vi "仪器参数设置.vi"(11 "仪器参数设置":T2 {"单位" items=["ug/L", "mg/L"]}) -> (3 "仪器参数设置输出":T1 {"单位" items=["ug/L", "mg/L"]})   [LabVIEW 2016, in "斯坦道CODMn.lvlib"]
uses:
  <vilib>/Utility/miscctls.llb/LVPointTypeDef.ctl
panel:
  in  "单位":enum16{"ug/L", "mg/L"}(ring)
  in  "标样校准时间":timestamp
  in  "二次多项式系数":dbl
  in  "线性相关系数":dbl
  in  "测量信号值":dbl
  in  "测量检出限":dbl
  in  "曲线斜率":dbl
  in  "曲线截距":dbl
  in  "空白校准时间":timestamp
  in  "消解时长":dbl
  in  "消解温度":dbl
  in  "测量间隔":dbl
  in  "测量精度":dbl
  in  "测量量程":dbl
  in  "取消":bool
  in  "确定":bool
  # "仪器参数设置"
  # "CODMn"
  # "监测参数"
  # "黑色框参数需要手动输入\n灰色框参数自动读取不需要手动输入"
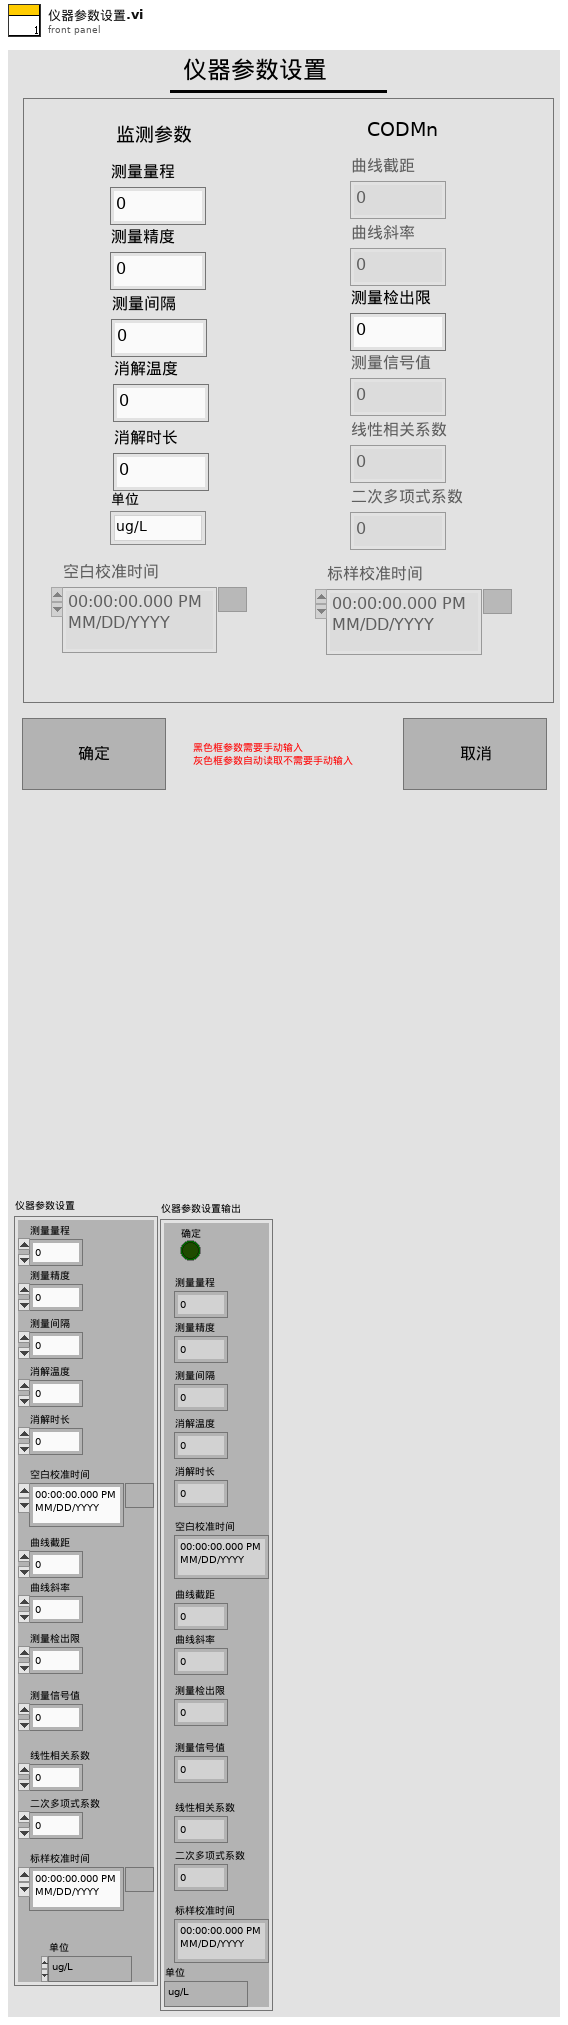
[diagram p1: front panel]
types:
  T1 = cluster{"确定":bool, "测量量程":dbl, "测量精度":dbl, "测量间隔":dbl, "消解温度":dbl, "消解时长":dbl, "空白校准时间":timestamp, "曲线截距":dbl, "曲线斜率":dbl, "测量检出限":dbl, "测量信号值":dbl, "线性相关系数":dbl, "二次多项式系数":dbl, "标样校准时间":timestamp, "单位":u16}
  T2 = cluster{"测量量程":dbl, "测量精度":dbl, "测量间隔":dbl, "消解温度":dbl, "消解时长":dbl, "空白校准时间":timestamp, "曲线截距":dbl, "曲线斜率":dbl, "测量检出限":dbl, "测量信号值":dbl, "线性相关系数":dbl, "二次多项式系数":dbl, "标样校准时间":timestamp, "单位":u16}
  T3 = typedef "LVPointTypeDef.ctl" = cluster{"Horizontal":i16, "Vertical":i16}
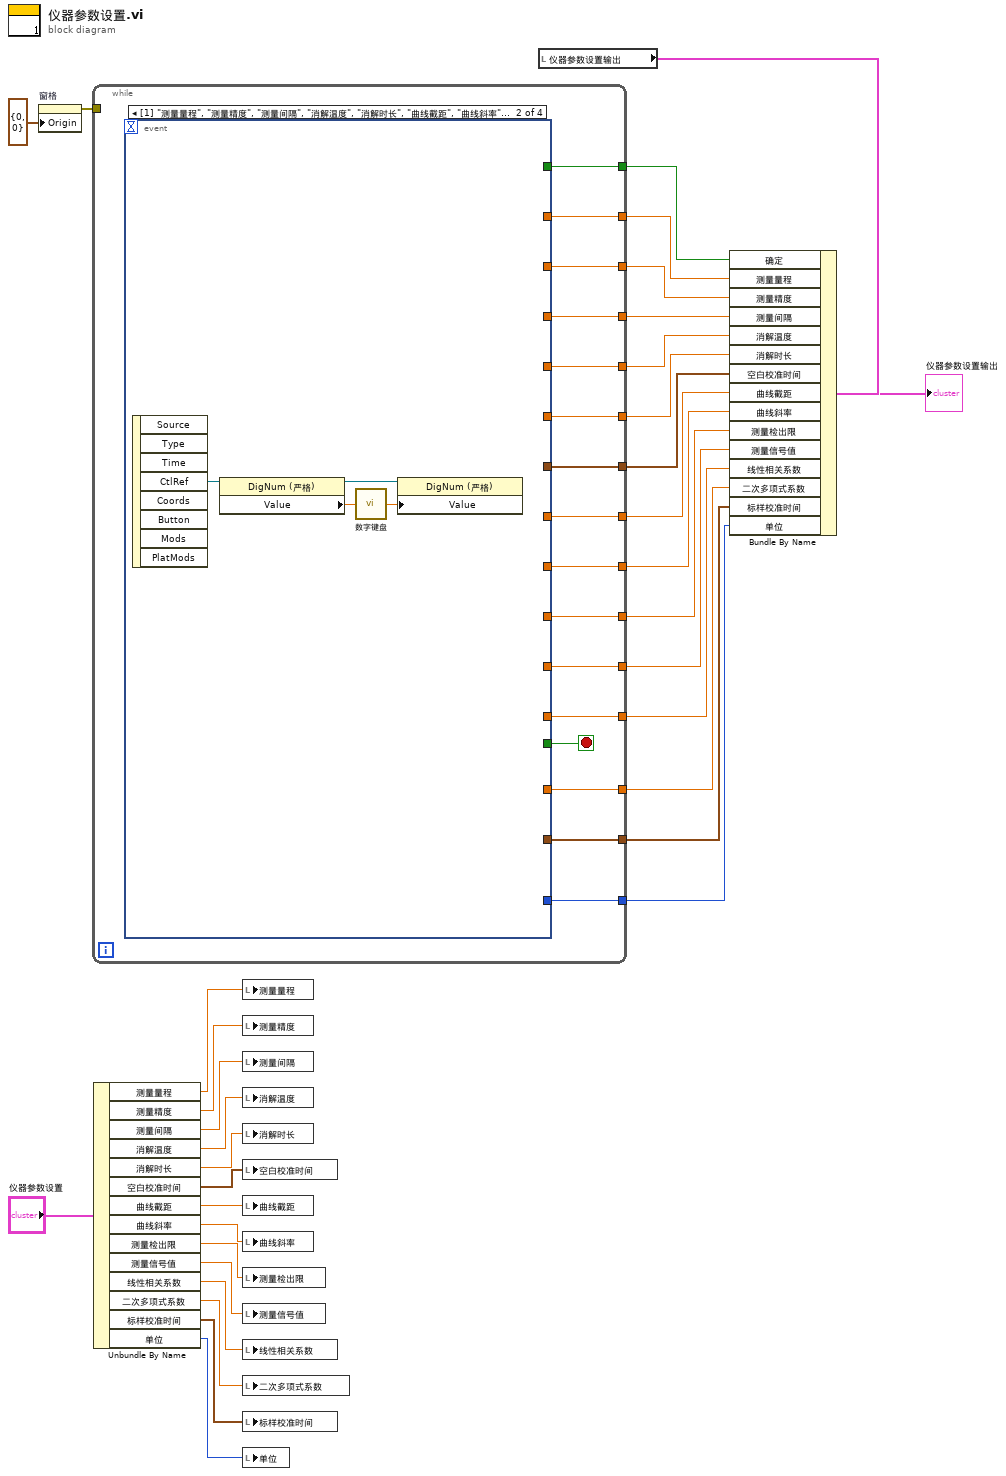
[diagram p0: block diagram]
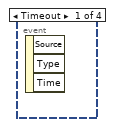
[diagram p2: hidden frame]
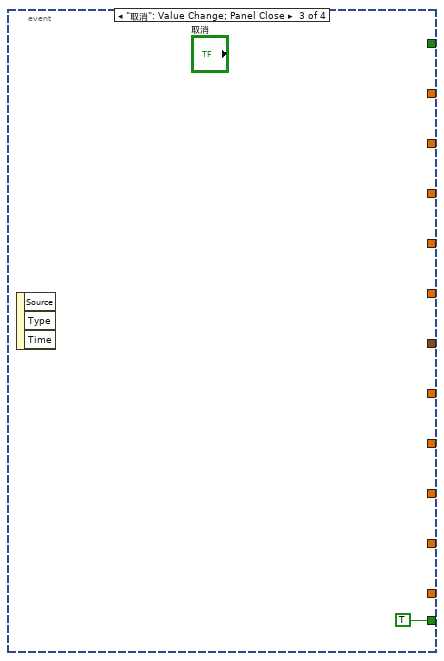
[diagram p3: hidden frame]
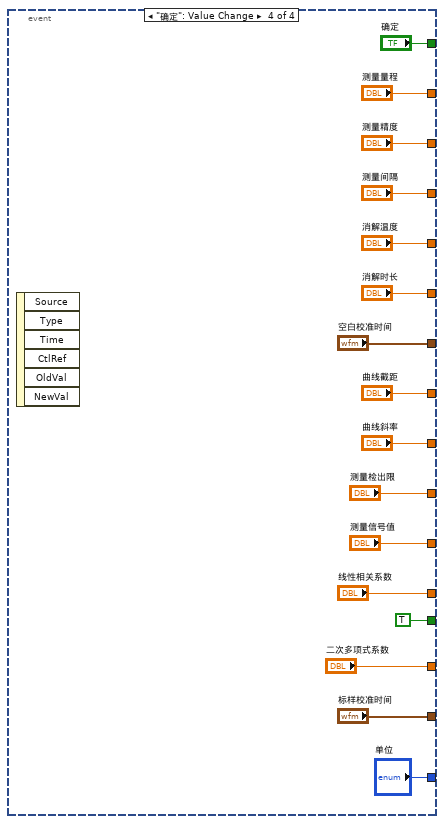
[diagram p4: hidden frame]
diagram:
  n1 = property on="窗格" class="Pane"("Origin"=T3 {"Horizontal"=0, "Vertical"=0} ("原点")) -> (error out=w33:errorcluster)  [unwired: 2 in, 1 out]
  n2 = while {
    tunnel: w33 -> [_]
    tunnel: [w49] -> w32
    tunnel: [w48] -> w28
    tunnel: [w47] -> w27
    tunnel: [w46] -> w26
    tunnel: [w45] -> w25
    tunnel: [w44] -> w24
    tunnel: [w43] -> w23
    tunnel: [w42] -> w22
    tunnel: [w41] -> w21
    tunnel: [w40] -> w20
    tunnel: [w39] -> w19
    tunnel: [w38] -> w18
    tunnel: [w37] -> w17
    tunnel: [w36] -> w16
    tunnel: [w35] -> w1
    stop <- w50 stop-if-true
    n3 = event shown="[1] \"测量量程\", \"测量精度\", \"测量间隔\", \"消解温度\", \"消解时长\", \"曲线截距\", \"曲线斜率\", \"测量检出限\", \"测量信号值\", \"线性相关系数\", \"二次多项式系数\": 鼠标按下" {
      selector: _ -> [_ _ _ _]
      dyn-events: _ -> [_ _ _ _]
      timeout: _ -> [_ _ _ _]
      tunnel: [_ _ TRUE TRUE] -> w50
      tunnel: [_ _ _ "确定"] -> w49
      tunnel: [_ _ _ "标样校准时间"] -> w48
      tunnel: [_ _ _ "二次多项式系数"] -> w47
      tunnel: [_ _ _ "线性相关系数"] -> w46
      tunnel: [_ _ _ "测量信号值"] -> w45
      tunnel: [_ _ _ "测量检出限"] -> w44
      tunnel: [_ _ _ "曲线斜率"] -> w43
      tunnel: [_ _ _ "曲线截距"] -> w42
      tunnel: [_ _ _ "空白校准时间"] -> w41
      tunnel: [_ _ _ "消解时长"] -> w40
      tunnel: [_ _ _ "消解温度"] -> w39
      tunnel: [_ _ _ "测量间隔"] -> w38
      tunnel: [_ _ _ "测量精度"] -> w37
      tunnel: [_ _ _ "测量量程"] -> w36
      tunnel: [_ _ _ "单位"] -> w35
      event Timeout {
        n4 = event-data() -> ()  [unwired: 1 in, 3 out]
      }
      event "测量量程", "测量精度", "测量间隔", "消解温度", "消解时长", "曲线截距", "曲线斜率", "测量检出限", "测量信号值", "线性相关系数", "二次多项式系数": Mouse Down {
        n5 = event-data() -> ("CtlRef"=w51:refnum<vi>)  [unwired: 1 in, 7 out]
        n6 = property class="DigNum (严格)"(reference=w51) -> (reference out=w53:refnum<vi>, "Value"=w54:dbl)  [unwired: 1 in, 1 out]
        n7 = call "数字键盘.vi"("OldNumber"=w54) -> ("NewNumber"=w52:sgl)
        n8 = property class="DigNum (严格)"(reference=w53, "Value"=w52) -> ()  [unwired: 1 in, 2 out]
      }
      event "取消": Value Change; Panel Close {
        n9 = event-data() -> ()  [unwired: 1 in, 3 out]
      }
      event "确定": Value Change {
        n10 = event-data() -> ()  [unwired: 1 in, 6 out]
      }
    }
  }
  n11 = Unbundle By Name("仪器参数设置") -> ("测量量程"=w15:dbl, "测量精度"=w14:dbl, "测量间隔"=w13:dbl, "消解温度"=w12:dbl, "消解时长"=w11:dbl, "空白校准时间"=w10:timestamp, "曲线截距"=w9:dbl, "曲线斜率"=w8:dbl, "测量检出限"=w7:dbl, "测量信号值"=w6:dbl, "线性相关系数"=w5:dbl, "二次多项式系数"=w4:dbl, "标样校准时间"=w3:timestamp, "单位"=w2:u16)
  n12 = local write "测量量程"(w15) -> ()
  n13 = local write "测量精度"(w14) -> ()
  n14 = local write "测量间隔"(w13) -> ()
  n15 = local write "消解温度"(w12) -> ()
  n16 = local write "消解时长"(w11) -> ()
  n17 = local write "空白校准时间"(w10) -> ()
  n18 = local write "曲线截距"(w9) -> ()
  n19 = local write "曲线斜率"(w8) -> ()
  n20 = local write "测量检出限"(w7) -> ()
  n21 = local write "测量信号值"(w6) -> ()
  n22 = local write "线性相关系数"(w5) -> ()
  n23 = local write "二次多项式系数"(w4) -> ()
  n24 = local write "标样校准时间"(w3) -> ()
  n25 = local write "单位"(w2) -> ()
  n26 = local read "仪器参数设置输出"() -> (w30:T1)
  n27 = Bundle By Name(cluster=w30, "确定"=w32, "测量量程"=w16, "测量精度"=w17, "测量间隔"=w18, "消解温度"=w19, "消解时长"=w20, "空白校准时间"=w21, "曲线截距"=w22, "曲线斜率"=w23, "测量检出限"=w24, "测量信号值"=w25, "线性相关系数"=w26, "二次多项式系数"=w27, "标样校准时间"=w28, "单位"=w1) -> (→"仪器参数设置输出":T1)
